vi "offlineInputSimulator.vi"(6 "ABORT":bool, 7 "Initial Timestamp":timestamp, 9 "Current Timestamp":timestamp, 10 "Waveform":waveform(dbl), 11 "Process_REF":string) -> (1 "Process Variable":dbl, 2 "Signal Out":dbl)   [LabVIEW 2018]
panel:
  out "Control Variable":dbl
  out "Boolean":bool
  out "Relative Time":dbl
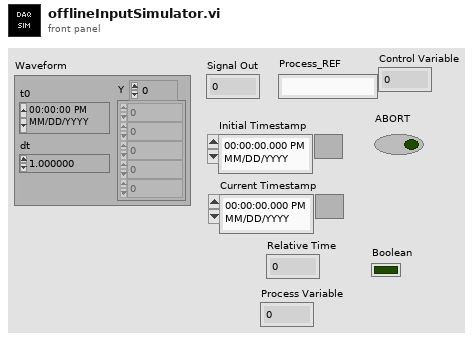
[diagram p1: front panel]
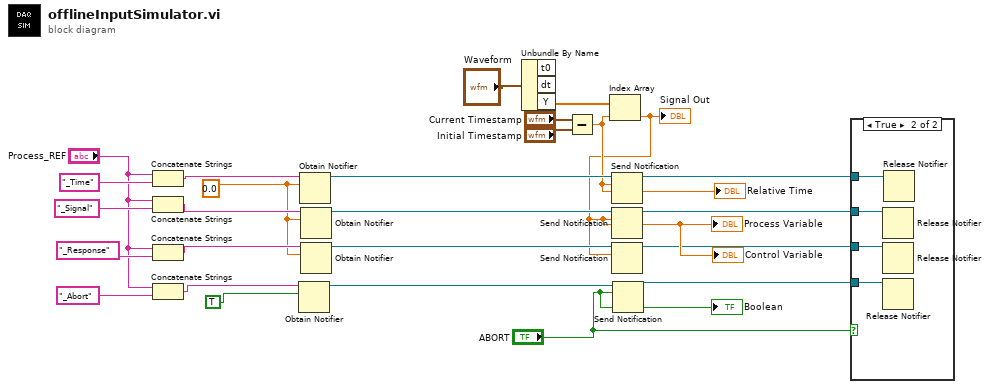
[diagram p0: block diagram]
diagram:
  w13 = 0.0
  n1 = Concatenate Strings("Process_REF", "_Time") -> (w14:string)
  n2 = Concatenate Strings("Process_REF", "_Signal") -> (w15:string)
  n3 = Concatenate Strings("Process_REF", "_Response") -> (w16:string)
  n4 = Concatenate Strings("Process_REF", "_Abort") -> (w17:string)
  n5 = Obtain Notifier(name (unnamed)=w17, notification data type=TRUE) -> (notifier out=w11:refnum<notifier>)  [unwired: 2 in, 2 out]
  n6 = Obtain Notifier(name (unnamed)=w14, notification data type=w13) -> (notifier out=w8:refnum<notifier>)  [unwired: 2 in, 2 out]
  n7 = Obtain Notifier(name (unnamed)=w15, notification data type=w13) -> (notifier out=w9:refnum<notifier>)  [unwired: 2 in, 2 out]
  n8 = Obtain Notifier(name (unnamed)=w16, notification data type=w13) -> (notifier out=w10:refnum<notifier>)  [unwired: 2 in, 2 out]
  n9 = Unbundle By Name("Waveform") -> ("Y"=w25:dbl[])  [unwired: 2 out]
  n10 = Subtract(x="Current Timestamp", y="Initial Timestamp") -> (x-y=w7:dbl)
  "Relative Time" <- w7
  n11 = Index Array(array=w25, index=w7) -> (element=w6:dbl)
  "Signal Out" <- w6
  "Process Variable" <- w6
  "Control Variable" <- w6
  n12 = Send Notification(notification=w7, notifier=w8) -> (notifier out=w1:refnum<notifier>)  [unwired: 1 in, 1 out]
  n13 = Send Notification(notification=w6, notifier=w9) -> (notifier out=w2:refnum<notifier>)  [unwired: 1 in, 1 out]
  n14 = Send Notification(notification=w6, notifier=w10) -> (notifier out=w3:refnum<notifier>)  [unwired: 1 in, 1 out]
  n15 = Send Notification(notification="ABORT", notifier=w11) -> (notifier out=w4:refnum<notifier>)  [unwired: 1 in, 1 out]
  n16 = case shown="True" "ABORT" {
    tunnel: w4 -> [_ w30]
    tunnel: w3 -> [_ w29]
    tunnel: w2 -> [_ w28]
    tunnel: w1 -> [_ w27]
    frame False {
    }
    frame True {
      n17 = Release Notifier(notifier=w28) -> ()  [unwired: 2 in, 3 out]
      n18 = Release Notifier(notifier=w29) -> ()  [unwired: 2 in, 3 out]
      n19 = Release Notifier(notifier=w30) -> ()  [unwired: 2 in, 3 out]
      n20 = Release Notifier(notifier=w27) -> ()  [unwired: 2 in, 3 out]
    }
  }
  "Boolean" <- "ABORT"
